vi "输入数据解析.vi"(0 "单个参数补充":dbl, 1 "从板号":dbl=1.0, 2 "主板二维码":string="BNET01", 3 "从板二维码":string="BNET01", 5 "主板引用":refnum<vi>, 7 "从板引用":refnum<vi>, 9 "主板选项":string="三级故障阀值", 11 "枚举":enum16{"主板", "从板"}(ring), 12 "快换":bool caption="快换写入") -> (4 "输出数组":dbl[][](array[numeric]), 6 "数组长度":dbl[](array[numeric]), 8 "循环次数":i32, 10 "命令":u32, 14 "名称":string[](array[string]), 15 "命令序号":u32[](array[numeric]))   [LabVIEW 2013] (continued)
                  disable-tunnel: [w8295 255 ("高字节1")] -> w8291
                  disable-tunnel: w8289 -> [w8293 _]
                  frame Disabled {
                    n3202 = Unbundle By Name(w8293) -> ("单组温度不均衡"=w8292:dbl)
                    n3203 = call "输入分辨率计算-EV05.vi"("1字节?"=TRUE, "数值"=w8292, "偏移量"=0.0, "分辨率"=1.0) -> ("高字节1"=w8295:dbl)  [unwired: 1 in, 6 out]
                  }
                  frame Enabled {
                  }
                }
                n3204 = Build Array(w8291) -> (w8290:i32[])
              }
              frame 12 {
                n3205 = Unbundle By Name(w8303) -> ("SOC过高"=w8302:dbl)
                n3206 = call "输入分辨率计算-EV05.vi"("1字节?"=FALSE, "数值"=w8302, "偏移量"=0.0, "分辨率"=0.1) -> ("低字节"=w8304:dbl, "高字节1"=w8305:dbl)  [unwired: 1 in, 5 out]
                n3207 = call "二进制解析-8.6.vi"("索引"=4, "数值"=w8305) -> ("低位子数组"=w8308:i32[])  [unwired: 3 out]
                n3208 = call "二进制解析-8.6.vi"("索引"=4, "数值"=w8304) -> ("低位子数组"=w8300:i32[], "高位子数组"=w8307:i32[])  [unwired: 2 out]
                n3209 = Insert Into Array(array=w8308, new element=w8307) -> (w8306:i32[])  [unwired: 1 in]
                n3210 = call "数值二进制转十进制-8.6.vi"("子数组"=w8306) -> ("十进制数值"=w8301:i32)  [unwired: 4 out]
                n3211 = disable-structure shown="启用" {
                  disable-tunnel: w8301 -> [w8316 _]
                  disable-tunnel: [w8316 255 ("高字节1")] -> w8299
                  disable-tunnel: [w8315 i32[] [] ("低位子数组 28")] -> _
                  disable-tunnel: w8300 -> [w8315 _]
                  frame Disabled {
                  }
                  frame Enabled {
                  }
                }
                n3212 = Build Array(w8299, w8299) -> (w8312:i32[])
              }
              frame 13 {
                # "SOC过低"
                n3213 = Unbundle By Name(w8324) -> ("SOC过低"=w8323:dbl)
                n3214 = call "输入分辨率计算-EV05.vi"("1字节?"=FALSE, "数值"=w8323, "偏移量"=0.0, "分辨率"=0.1) -> ("低字节"=w8321:dbl, "高字节1"=w8322:dbl)  [unwired: 1 in, 5 out]
                n3215 = call "二进制解析-8.6.vi"("索引"=4, "数值"=w8322) -> ("低位子数组"=w8320:i32[])  [unwired: 3 out]
                n3216 = disable-structure shown="启用" {
                  disable-tunnel: w8321 -> [w8331 _]
                  disable-tunnel: [w8331 255 ("高字节1")] -> w8319
                  disable-tunnel: w8320 -> [w8330 _]
                  disable-tunnel: [w8330 i32[] [] ("低位子数组")] -> _
                  frame Disabled {
                    (unwired) i32[] [] ("低位子数组 4")
                  }
                  frame Enabled {
                  }
                }
                n3217 = Build Array(w8319, w8319) -> (w8327:i32[])
              }
              frame 14 {
                # "内阻过大"
                n3218 = disable-structure shown="启用" {
                  disable-tunnel: w8336 -> [w8341 _]
                  disable-tunnel: [w8337 255 ("高字节1")] -> w8334
                  frame Disabled {
                    n3219 = Unbundle By Name(w8341) -> ("内阻过大"=w8340:dbl)
                    n3220 = call "输入分辨率计算-EV05.vi"("1字节?"=TRUE, "数值"=w8340, "分辨率"=0.1) -> ("高字节1"=w8337:dbl)  [unwired: 2 in, 6 out]
                  }
                  frame Enabled {
                  }
                }
                n3221 = Build Array(w8334) -> (w8335:i32[])
              }
              frame 15 {
                # "极柱温度过高"
                n3222 = disable-structure shown="启用" {
                  disable-tunnel: w8345 -> [w8351 _]
                  disable-tunnel: [w8347 255 ("高字节1")] -> w8343
                  frame Disabled {
                    n3223 = Unbundle By Name(w8351) -> ("极柱温度过高"=w8350:dbl)
                    n3224 = call "输入分辨率计算-EV05.vi"("1字节?"=TRUE, "数值"=w8350, "偏移量"=-40.0, "分辨率"=1.0) -> ("高字节1"=w8347:dbl)  [unwired: 1 in, 6 out]
                  }
                  frame Enabled {
                  }
                }
                n3225 = Build Array(w8343) -> (w8344:i32[])
              }
              frame 16 {
                # "SOH过低"
                n3226 = disable-structure shown="启用" {
                  disable-tunnel: [w8368 w8376] -> w8355
                  disable-tunnel: w8354 -> [w8365 _]
                  disable-tunnel: [w8357 w8376] -> w8353
                  frame Disabled {
                    n3227 = Unbundle By Name(w8365) -> ("SOH过低"=w8364:dbl)
                    n3228 = call "输入分辨率计算-EV05.vi"("1字节?"=FALSE, "数值"=w8364, "偏移量"=0.0, "分辨率"=0.1) -> ("低字节"=w8366:dbl, "高字节1"=w8367:dbl)  [unwired: 1 in, 5 out]
                    n3229 = call "二进制解析-8.6.vi"("索引"=4, "数值"=w8367) -> ("低位子数组"=w8370:i32[])  [unwired: 3 out]
                    n3230 = call "二进制解析-8.6.vi"("索引"=4, "数值"=w8366) -> ("低位子数组"=w8359:i32[], "高位子数组"=w8369:i32[])  [unwired: 2 out]
                    n3231 = call "二进制解析-8.6.vi"("索引"=4, "数值"=0) -> ("低位子数组"=w8360:i32[])  [unwired: 3 out]
                    n3232 = Insert Into Array(array=w8370, new element=w8369) -> (w8363:i32[])  [unwired: 1 in]
                    n3233 = Insert Into Array(array=w8359, new element=w8360) -> (w8358:i32[])  [unwired: 1 in]
                    n3234 = call "数值二进制转十进制-8.6.vi"("子数组"=w8363) -> ("十进制数值"=w8368:i32)  [unwired: 4 out]
                    n3235 = call "数值二进制转十进制-8.6.vi"("子数组"=w8358) -> ("十进制数值"=w8357:i32)  [unwired: 4 out]
                  }
                  frame Enabled {
                    w8376 = 255 ("高字节1")
                  }
                }
                n3236 = Build Array(w8355, w8353) -> (w8356:i32[])
              }
            }
            n3237 = Insert Into Array(array=w8161, new element=w8162) -> (w8160:dbl[])  [unwired: 1 in]
          }
          n3238 = Build Array(w8157) -> (w8156:dbl[][])
          n3239 = Build Array("二级故障阀值") -> (w8147:string[])
        }
        frame "放电电流过高(3)" {
          n3240 = Unbundle By Name(w8382) -> ("一级故障 3"=w8383:refnum<vi>)
          n3241 = property class="Clust (严格)"(reference=w8383) -> ("Value"=w8381:T4)  [unwired: 1 in, 2 out]
          n3242 = for {
            N: 17 -> [_]
            tunnel: w8381 -> [w8393]
            shift-right: [w8390] -> w8387
            shift-left: dbl[] [] -> [w8391]
            i -> [w8394]
            n3243 = case shown="14" w8394 {
              tunnel: w8393 -> [w8395 w8406 w8417 w8427 w8437 w8447 w8459 w8471 w8483 w8495 w8507 w8519 w8533 w8554 w8566 w8575 w8584]
              tunnel: [w8396 w8407 w8418 w8428 w8438 w8449 w8461 w8473 w8485 w8497 w8509 w8520 w8542 w8557 w8565 w8574 w8586] -> w8392
              frame 0, Default {
                # "总电压过高"
                n3244 = disable-structure shown="启用" {
                  disable-tunnel: [w8402 w8405] -> w8398
                  disable-tunnel: [w8401 w8405] -> w8397
                  disable-tunnel: w8395 -> [w8400 _]
                  frame Disabled {
                    n3245 = Unbundle By Name(w8400) -> ("总电压过高"=w8399:dbl)
                    n3246 = call "输入分辨率计算-EV05.vi"("1字节?"=FALSE, "数值"=w8399, "分辨率"=0.1) -> ("低字节"=w8402:dbl, "高字节1"=w8401:dbl)  [unwired: 2 in, 5 out]
                  }
                  frame Enabled {
                    w8405 = 255 ("高字节1")
                  }
                }
                n3247 = Build Array(w8397, w8398) -> (w8396:i32[])
              }
              frame 1 {
                # "总电压过低"
                n3248 = disable-structure shown="启用" {
                  disable-tunnel: [w8413 w8416] -> w8409
                  disable-tunnel: [w8412 w8416] -> w8408
                  disable-tunnel: w8406 -> [w8411 _]
                  frame Disabled {
                    n3249 = Unbundle By Name(w8411) -> ("总电压过低"=w8410:dbl)
                    n3250 = call "输入分辨率计算-EV05.vi"("1字节?"=FALSE, "数值"=w8410, "分辨率"=0.1) -> ("低字节"=w8413:dbl, "高字节1"=w8412:dbl)  [unwired: 2 in, 5 out]
                  }
                  frame Enabled {
                    w8416 = 255 ("高字节1")
                  }
                }
                n3251 = Build Array(w8408, w8409) -> (w8407:i32[])
              }
              frame 2 {
                # "温度过高"
                n3252 = disable-structure shown="启用" {
                  disable-tunnel: [w8423 255 ("高字节1")] -> w8419
                  disable-tunnel: w8417 -> [w8421 _]
                  frame Disabled {
                    n3253 = Unbundle By Name(w8421) -> ("温度过高"=w8420:dbl)
                    n3254 = call "输入分辨率计算-EV05.vi"("1字节?"=TRUE, "数值"=w8420, "偏移量"=-40.0, "分辨率"=1.0) -> ("高字节1"=w8423:dbl)  [unwired: 1 in, 6 out]
                  }
                  frame Enabled {
                  }
                }
                n3255 = Build Array(w8419) -> (w8418:i32[])
              }
              frame 3 {
                # "温度过低"
                n3256 = disable-structure shown="启用" {
                  disable-tunnel: [w8433 255 ("高字节1")] -> w8429
                  disable-tunnel: w8427 -> [w8431 _]
                  frame Disabled {
                    n3257 = Unbundle By Name(w8431) -> ("温度过低"=w8430:dbl)
                    n3258 = call "输入分辨率计算-EV05.vi"("1字节?"=TRUE, "数值"=w8430, "偏移量"=-40.0, "分辨率"=1.0) -> ("高字节1"=w8433:dbl)  [unwired: 1 in, 6 out]
                  }
                  frame Enabled {
                  }
                }
                n3259 = Build Array(w8429) -> (w8428:i32[])
              }
              frame 4 {
                # "整组温度不均衡"
                n3260 = disable-structure shown="启用" {
                  disable-tunnel: [w8443 255 ("高字节1")] -> w8439
                  disable-tunnel: w8437 -> [w8441 _]
                  frame Disabled {
                    n3261 = Unbundle By Name(w8441) -> ("整组温度不均衡"=w8440:dbl)
                    n3262 = call "输入分辨率计算-EV05.vi"("1字节?"=TRUE, "数值"=w8440, "偏移量"=0.0, "分辨率"=1.0) -> ("高字节1"=w8443:dbl)  [unwired: 1 in, 6 out]
                  }
                  frame Enabled {
                  }
                }
                n3263 = Build Array(w8439) -> (w8438:i32[])
              }
              frame 5 {
                # "单组电压不均衡"
                n3264 = disable-structure shown="启用" {
                  disable-tunnel: [w8455 w8458] -> w8450
                  disable-tunnel: [w8453 w8458] -> w8448
                  disable-tunnel: w8447 -> [w8452 _]
                  frame Disabled {
                    n3265 = Unbundle By Name(w8452) -> ("单组电压不均衡"=w8451:dbl)
                    n3266 = call "输入分辨率计算-EV05.vi"("1字节?"=FALSE, "数值"=w8451, "偏移量"=0.0, "分辨率"=0.001) -> ("低字节"=w8453:dbl, "高字节1"=w8455:dbl)  [unwired: 1 in, 5 out]
                  }
                  frame Enabled {
                    w8458 = 255 ("高字节1")
                  }
                }
                n3267 = Build Array(w8450, w8448) -> (w8449:i32[])
              }
              frame 6 {
                # "整组电压不均衡"
                n3268 = disable-structure shown="启用" {
                  disable-tunnel: [w8467 w8470] -> w8462
                  disable-tunnel: [w8465 w8470] -> w8460
                  disable-tunnel: w8459 -> [w8464 _]
                  frame Disabled {
                    n3269 = Unbundle By Name(w8464) -> ("整组电压不均衡"=w8463:dbl)
                    n3270 = call "输入分辨率计算-EV05.vi"("1字节?"=FALSE, "数值"=w8463, "偏移量"=0.0, "分辨率"=0.001) -> ("低字节"=w8465:dbl, "高字节1"=w8467:dbl)  [unwired: 1 in, 5 out]
                  }
                  frame Enabled {
                    w8470 = 255 ("高字节1")
                  }
                }
                n3271 = Build Array(w8462, w8460) -> (w8461:i32[])
              }
              frame 7 {
                # "单体电压过高"
                n3272 = disable-structure shown="启用" {
                  disable-tunnel: [w8479 w8482] -> w8474
                  disable-tunnel: [w8477 w8482] -> w8472
                  disable-tunnel: w8471 -> [w8476 _]
                  frame Disabled {
                    n3273 = Unbundle By Name(w8476) -> ("单体电压过高"=w8475:dbl)
                    n3274 = call "输入分辨率计算-EV05.vi"("1字节?"=FALSE, "数值"=w8475, "偏移量"=0.0, "分辨率"=0.001) -> ("低字节"=w8477:dbl, "高字节1"=w8479:dbl)  [unwired: 1 in, 5 out]
                  }
                  frame Enabled {
                    w8482 = 255 ("高字节1")
                  }
                }
                n3275 = Build Array(w8474, w8472) -> (w8473:i32[])
              }
              frame 8 {
                # "单体电压过低"
                n3276 = disable-structure shown="启用" {
                  disable-tunnel: [w8491 w8494] -> w8486
                  disable-tunnel: [w8489 w8494] -> w8484
                  disable-tunnel: w8483 -> [w8488 _]
                  frame Disabled {
                    n3277 = Unbundle By Name(w8488) -> ("单体电压过低"=w8487:dbl)
                    n3278 = call "输入分辨率计算-EV05.vi"("1字节?"=FALSE, "数值"=w8487, "偏移量"=0.0, "分辨率"=0.001) -> ("低字节"=w8489:dbl, "高字节1"=w8491:dbl)  [unwired: 1 in, 5 out]
                  }
                  frame Enabled {
                    w8494 = 255 ("高字节1")
                  }
                }
                n3279 = Build Array(w8486, w8484) -> (w8485:i32[])
              }
              frame 9 {
                # "充电电流过高"
                n3280 = disable-structure shown="启用" {
                  disable-tunnel: [w8503 w8506] -> w8498
                  disable-tunnel: [w8501 w8506] -> w8496
                  disable-tunnel: w8495 -> [w8500 _]
                  frame Disabled {
                    n3281 = Unbundle By Name(w8500) -> ("充电电流过高"=w8499:dbl)
                    n3282 = call "输入分辨率计算-EV05.vi"("1字节?"=FALSE, "数值"=w8499, "偏移量"=-3000.0, "分辨率"=0.1) -> ("低字节"=w8501:dbl, "高字节1"=w8503:dbl)  [unwired: 1 in, 5 out]
                  }
                  frame Enabled {
                    w8506 = 255 ("高字节1")
                  }
                }
                n3283 = Build Array(w8498, w8496) -> (w8497:i32[])
              }
              frame 10 {
                # "放电电流过高"
                n3284 = disable-structure shown="启用" {
                  disable-tunnel: [w8515 w8518] -> w8510
                  disable-tunnel: [w8513 w8518] -> w8508
                  disable-tunnel: w8507 -> [w8512 _]
                  frame Enabled {
                    n3285 = Unbundle By Name(w8512) -> ("放电电流过高"=w8511:dbl)
                    n3286 = call "输入分辨率计算-EV05.vi"("1字节?"=FALSE, "数值"=w8511, "偏移量"=0.0, "分辨率"=0.1) -> ("低字节"=w8513:dbl, "高字节1"=w8515:dbl)  [unwired: 1 in, 5 out]
                  }
                  frame Disabled {
                    w8518 = 255 ("高字节1")
                  }
                }
                n3287 = Build Array(w8510, w8508) -> (w8509:dbl[])
              }
              frame 11 {
                # "单组温度不均衡"
                n3288 = disable-structure shown="启用" {
                  disable-tunnel: [w8525 255 ("高字节1")] -> w8521
                  disable-tunnel: w8519 -> [w8523 _]
                  frame Disabled {
                    n3289 = Unbundle By Name(w8523) -> ("单组温度不均衡"=w8522:dbl)
                    n3290 = call "输入分辨率计算-EV05.vi"("1字节?"=TRUE, "数值"=w8522, "偏移量"=0.0, "分辨率"=1.0) -> ("高字节1"=w8525:dbl)  [unwired: 1 in, 6 out]
                  }
                  frame Enabled {
                  }
                }
                n3291 = Build Array(w8521) -> (w8520:i32[])
              }
              frame 12 {
                # "SOC过高"
                n3292 = Unbundle By Name(w8533) -> ("SOC过高"=w8532:dbl)
                n3293 = call "输入分辨率计算-EV05.vi"("1字节?"=FALSE, "数值"=w8532, "偏移量"=0.0, "分辨率"=0.1) -> ("低字节"=w8534:dbl, "高字节1"=w8535:dbl)  [unwired: 1 in, 5 out]
                n3294 = call "二进制解析-8.6.vi"("索引"=4, "数值"=w8535) -> ("低位子数组"=w8538:i32[])  [unwired: 3 out]
                n3295 = call "二进制解析-8.6.vi"("索引"=4, "数值"=w8534) -> ("低位子数组"=w8530:i32[], "高位子数组"=w8537:i32[])  [unwired: 2 out]
                n3296 = Insert Into Array(array=w8538, new element=w8537) -> (w8536:i32[])  [unwired: 1 in]
                n3297 = call "数值二进制转十进制-8.6.vi"("子数组"=w8536) -> ("十进制数值"=w8531:i32)  [unwired: 4 out]
                n3298 = disable-structure shown="启用" {
                  disable-tunnel: w8531 -> [w8546 _]
                  disable-tunnel: [w8546 255 ("高字节1")] -> w8529
                  disable-tunnel: [w8545 i32[] [] ("低位子数组 28")] -> _
                  disable-tunnel: w8530 -> [w8545 _]
                  frame Disabled {
                  }
                  frame Enabled {
                  }
                }
                n3299 = Build Array(w8529, w8529) -> (w8542:i32[])
              }
              frame 13 {
                # "SOC过低"
                n3300 = Unbundle By Name(w8554) -> ("SOC过低"=w8553:dbl)
                n3301 = call "输入分辨率计算-EV05.vi"("1字节?"=FALSE, "数值"=w8553, "偏移量"=0.0, "分辨率"=0.1) -> ("低字节"=w8551:dbl, "高字节1"=w8552:dbl)  [unwired: 1 in, 5 out]
                n3302 = call "二进制解析-8.6.vi"("索引"=4, "数值"=w8552) -> ("低位子数组"=w8550:i32[])  [unwired: 3 out]
                n3303 = disable-structure shown="启用" {
                  disable-tunnel: w8551 -> [w8561 _]
                  disable-tunnel: [w8561 255 ("高字节1")] -> w8549
                  disable-tunnel: w8550 -> [w8560 _]
                  disable-tunnel: [w8560 i32[] [] ("低位子数组")] -> _
                  frame Disabled {
                    (unwired) i32[] [] ("低位子数组 4")
                  }
                  frame Enabled {
                  }
                }
                n3304 = Build Array(w8549, w8549) -> (w8557:i32[])
              }
              frame 14 {
                # "内阻过大"
                n3305 = disable-structure shown="启用" {
                  disable-tunnel: w8566 -> [w8571 _]
                  disable-tunnel: [w8567 255 ("高字节1")] -> w8564
                  frame Disabled {
                    n3306 = Unbundle By Name(w8571) -> ("内阻过大"=w8570:dbl)
                    n3307 = call "输入分辨率计算-EV05.vi"("1字节?"=TRUE, "数值"=w8570, "分辨率"=0.1) -> ("高字节1"=w8567:dbl)  [unwired: 2 in, 6 out]
                  }
                  frame Enabled {
                  }
                }
                n3308 = Build Array(w8564) -> (w8565:i32[])
              }
              frame 15 {
                # "极柱温度过高"
                n3309 = disable-structure shown="启用" {
                  disable-tunnel: w8575 -> [w8581 _]
                  disable-tunnel: [w8577 255 ("高字节1")] -> w8573
                  frame Disabled {
                    n3310 = Unbundle By Name(w8581) -> ("极柱温度过高"=w8580:dbl)
                    n3311 = call "输入分辨率计算-EV05.vi"("1字节?"=TRUE, "数值"=w8580, "偏移量"=-40.0, "分辨率"=1.0) -> ("高字节1"=w8577:dbl)  [unwired: 1 in, 6 out]
                  }
                  frame Enabled {
                  }
                }
                n3312 = Build Array(w8573) -> (w8574:i32[])
              }
              frame 16 {
                # "SOH过低"
                n3313 = disable-structure shown="启用" {
                  disable-tunnel: [w8598 w8606] -> w8585
                  disable-tunnel: w8584 -> [w8595 _]
                  disable-tunnel: [w8587 w8606] -> w8583
                  frame Disabled {
                    n3314 = Unbundle By Name(w8595) -> ("SOH过低"=w8594:dbl)
                    n3315 = call "输入分辨率计算-EV05.vi"("1字节?"=FALSE, "数值"=w8594, "偏移量"=0.0, "分辨率"=0.1) -> ("低字节"=w8596:dbl, "高字节1"=w8597:dbl)  [unwired: 1 in, 5 out]
                    n3316 = call "二进制解析-8.6.vi"("索引"=4, "数值"=w8597) -> ("低位子数组"=w8600:i32[])  [unwired: 3 out]
                    n3317 = call "二进制解析-8.6.vi"("索引"=4, "数值"=w8596) -> ("低位子数组"=w8589:i32[], "高位子数组"=w8599:i32[])  [unwired: 2 out]
                    n3318 = call "二进制解析-8.6.vi"("索引"=4, "数值"=0) -> ("低位子数组"=w8590:i32[])  [unwired: 3 out]
                    n3319 = Insert Into Array(array=w8600, new element=w8599) -> (w8593:i32[])  [unwired: 1 in]
                    n3320 = Insert Into Array(array=w8589, new element=w8590) -> (w8588:i32[])  [unwired: 1 in]
                    n3321 = call "数值二进制转十进制-8.6.vi"("子数组"=w8593) -> ("十进制数值"=w8598:i32)  [unwired: 4 out]
                    n3322 = call "数值二进制转十进制-8.6.vi"("子数组"=w8588) -> ("十进制数值"=w8587:i32)  [unwired: 4 out]
                  }
                  frame Enabled {
                    w8606 = 255 ("高字节1")
                  }
                }
                n3323 = Build Array(w8585, w8583) -> (w8586:i32[])
              }
            }
            n3324 = Insert Into Array(array=w8391, new element=w8392) -> (w8390:dbl[])  [unwired: 1 in]
          }
          n3325 = Build Array(w8387) -> (w8386:dbl[][])
          n3326 = Build Array("三级故障阀值") -> (w8377:string[])
        }
        frame "单组温度不均衡" {
          n3327 = Unbundle By Name(w8612) -> ("一级故障"=w8613:refnum<vi>)
          n3328 = property class="Clust (严格)"(reference=w8613) -> ("Value"=w8611:T4)  [unwired: 1 in, 2 out]
          n3329 = for {
            N: 17 -> [_]
            tunnel: w8611 -> [w8623]
            shift-right: [w8620] -> w8617
            shift-left: dbl[] [] -> [w8621]
            i -> [w8624]
            n3330 = case shown="11" w8624 {
              tunnel: w8623 -> [w8625 w8636 w8647 w8657 w8667 w8677 w8689 w8701 w8713 w8725 w8737 w8749 w8762 w8783 w8795 w8804 w8813]
              tunnel: [w8626 w8637 w8648 w8658 w8668 w8679 w8691 w8703 w8715 w8727 w8739 w8750 w8771 w8786 w8794 w8803 w8815] -> w8622
              frame 0, Default {
                # "总电压过高"
                n3331 = disable-structure shown="启用" {
                  disable-tunnel: [w8632 w8635] -> w8628
                  disable-tunnel: [w8631 w8635] -> w8627
                  disable-tunnel: w8625 -> [w8630 _]
                  frame Disabled {
                    n3332 = Unbundle By Name(w8630) -> ("总电压过高"=w8629:dbl)
                    n3333 = call "输入分辨率计算-EV05.vi"("1字节?"=FALSE, "数值"=w8629, "分辨率"=0.1) -> ("低字节"=w8632:dbl, "高字节1"=w8631:dbl)  [unwired: 2 in, 5 out]
                  }
                  frame Enabled {
                    w8635 = 255 ("高字节1")
                  }
                }
                n3334 = Build Array(w8627, w8628) -> (w8626:i32[])
              }
              frame 1 {
                # "总电压过低"
                n3335 = disable-structure shown="启用" {
                  disable-tunnel: [w8643 w8646] -> w8639
                  disable-tunnel: [w8642 w8646] -> w8638
                  disable-tunnel: w8636 -> [w8641 _]
                  frame Disabled {
                    n3336 = Unbundle By Name(w8641) -> ("总电压过低"=w8640:dbl)
                    n3337 = call "输入分辨率计算-EV05.vi"("1字节?"=FALSE, "数值"=w8640, "分辨率"=0.1) -> ("低字节"=w8643:dbl, "高字节1"=w8642:dbl)  [unwired: 2 in, 5 out]
                  }
                  frame Enabled {
                    w8646 = 255 ("高字节1")
                  }
                }
                n3338 = Build Array(w8638, w8639) -> (w8637:i32[])
              }
              frame 2 {
                # "温度过高"
                n3339 = disable-structure shown="启用" {
                  disable-tunnel: [w8653 255 ("高字节1")] -> w8649
                  disable-tunnel: w8647 -> [w8651 _]
                  frame Disabled {
                    n3340 = Unbundle By Name(w8651) -> ("温度过高"=w8650:dbl)
                    n3341 = call "输入分辨率计算-EV05.vi"("1字节?"=TRUE, "数值"=w8650, "偏移量"=-40.0, "分辨率"=1.0) -> ("高字节1"=w8653:dbl)  [unwired: 1 in, 6 out]
                  }
                  frame Enabled {
                  }
                }
                n3342 = Build Array(w8649) -> (w8648:i32[])
              }
              frame 3 {
                # "温度过低"
                n3343 = disable-structure shown="启用" {
                  disable-tunnel: [w8663 255 ("高字节1")] -> w8659
                  disable-tunnel: w8657 -> [w8661 _]
                  frame Disabled {
                    n3344 = Unbundle By Name(w8661) -> ("温度过低"=w8660:dbl)
                    n3345 = call "输入分辨率计算-EV05.vi"("1字节?"=TRUE, "数值"=w8660, "偏移量"=-40.0, "分辨率"=1.0) -> ("高字节1"=w8663:dbl)  [unwired: 1 in, 6 out]
                  }
                  frame Enabled {
                  }
                }
                n3346 = Build Array(w8659) -> (w8658:i32[])
              }
              frame 4 {
                # "整组温度不均衡"
                n3347 = disable-structure shown="启用" {
                  disable-tunnel: [w8673 255 ("高字节1")] -> w8669
                  disable-tunnel: w8667 -> [w8671 _]
                  frame Disabled {
                    n3348 = Unbundle By Name(w8671) -> ("整组温度不均衡"=w8670:dbl)
                    n3349 = call "输入分辨率计算-EV05.vi"("1字节?"=TRUE, "数值"=w8670, "偏移量"=0.0, "分辨率"=1.0) -> ("高字节1"=w8673:dbl)  [unwired: 1 in, 6 out]
                  }
                  frame Enabled {
                  }
                }
                n3350 = Build Array(w8669) -> (w8668:i32[])
              }
              frame 5 {
                # "单组电压不均衡"
                n3351 = disable-structure shown="启用" {
                  disable-tunnel: [w8685 w8688] -> w8680
                  disable-tunnel: [w8683 w8688] -> w8678
                  disable-tunnel: w8677 -> [w8682 _]
                  frame Disabled {
                    n3352 = Unbundle By Name(w8682) -> ("单组电压不均衡"=w8681:dbl)
                    n3353 = call "输入分辨率计算-EV05.vi"("1字节?"=FALSE, "数值"=w8681, "偏移量"=0.0, "分辨率"=0.001) -> ("低字节"=w8683:dbl, "高字节1"=w8685:dbl)  [unwired: 1 in, 5 out]
                  }
                  frame Enabled {
                    w8688 = 255 ("高字节1")
                  }
                }
                n3354 = Build Array(w8680, w8678) -> (w8679:i32[])
              }
              frame 6 {
                # "整组电压不均衡"
                n3355 = disable-structure shown="启用" {
                  disable-tunnel: [w8697 w8700] -> w8692
                  disable-tunnel: [w8695 w8700] -> w8690
                  disable-tunnel: w8689 -> [w8694 _]
                  frame Disabled {
                    n3356 = Unbundle By Name(w8694) -> ("整组电压不均衡"=w8693:dbl)
                    n3357 = call "输入分辨率计算-EV05.vi"("1字节?"=FALSE, "数值"=w8693, "偏移量"=0.0, "分辨率"=0.001) -> ("低字节"=w8695:dbl, "高字节1"=w8697:dbl)  [unwired: 1 in, 5 out]
                  }
                  frame Enabled {
                    w8700 = 255 ("高字节1")
                  }
                }
                n3358 = Build Array(w8692, w8690) -> (w8691:i32[])
              }
              frame 7 {
                # "单体电压过高"
                n3359 = disable-structure shown="启用" {
                  disable-tunnel: [w8709 w8712] -> w8704
                  disable-tunnel: [w8707 w8712] -> w8702
                  disable-tunnel: w8701 -> [w8706 _]
                  frame Disabled {
                    n3360 = Unbundle By Name(w8706) -> ("单体电压过高"=w8705:dbl)
                    n3361 = call "输入分辨率计算-EV05.vi"("1字节?"=FALSE, "数值"=w8705, "偏移量"=0.0, "分辨率"=0.001) -> ("低字节"=w8707:dbl, "高字节1"=w8709:dbl)  [unwired: 1 in, 5 out]
                  }
                  frame Enabled {
                    w8712 = 255 ("高字节1")
                  }
                }
                n3362 = Build Array(w8704, w8702) -> (w8703:i32[])
              }
              frame 8 {
                # "单体电压过低"
                n3363 = disable-structure shown="启用" {
                  disable-tunnel: [w8721 w8724] -> w8716
                  disable-tunnel: [w8719 w8724] -> w8714
                  disable-tunnel: w8713 -> [w8718 _]
                  frame Disabled {
                    n3364 = Unbundle By Name(w8718) -> ("单体电压过低"=w8717:dbl)
                    n3365 = call "输入分辨率计算-EV05.vi"("1字节?"=FALSE, "数值"=w8717, "偏移量"=0.0, "分辨率"=0.001) -> ("低字节"=w8719:dbl, "高字节1"=w8721:dbl)  [unwired: 1 in, 5 out]
                  }
                  frame Enabled {
                    w8724 = 255 ("高字节1")
                  }
                }
                n3366 = Build Array(w8716, w8714) -> (w8715:i32[])
              }
              frame 9 {
                # "充电电流过高"
                n3367 = disable-structure shown="启用" {
                  disable-tunnel: [w8733 w8736] -> w8728
                  disable-tunnel: [w8731 w8736] -> w8726
                  disable-tunnel: w8725 -> [w8730 _]
                  frame Disabled {
                    n3368 = Unbundle By Name(w8730) -> ("充电电流过高"=w8729:dbl)
                    n3369 = call "输入分辨率计算-EV05.vi"("1字节?"=FALSE, "数值"=w8729, "偏移量"=-3000.0, "分辨率"=0.1) -> ("低字节"=w8731:dbl, "高字节1"=w8733:dbl)  [unwired: 1 in, 5 out]
                  }
                  frame Enabled {
                    w8736 = 255 ("高字节1")
                  }
                }
                n3370 = Build Array(w8728, w8726) -> (w8727:i32[])
              }
              frame 10 {
                # "放电电流过高"
                n3371 = disable-structure shown="启用" {
                  disable-tunnel: [w8745 w8748] -> w8740
                  disable-tunnel: [w8743 w8748] -> w8738
                  disable-tunnel: w8737 -> [w8742 _]
                  frame Disabled {
                    n3372 = Unbundle By Name(w8742) -> ("放电电流过高"=w8741:dbl)
                    n3373 = call "输入分辨率计算-EV05.vi"("1字节?"=FALSE, "数值"=w8741, "偏移量"=-3000.0, "分辨率"=0.1) -> ("低字节"=w8743:dbl, "高字节1"=w8745:dbl)  [unwired: 1 in, 5 out]
                  }
                  frame Enabled {
                    w8748 = 255 ("高字节1")
                  }
                }
                n3374 = Build Array(w8740, w8738) -> (w8739:i32[])
              }
              frame 11 {
                # "单组温度不均衡"
                n3375 = disable-structure shown="启用" {
                  disable-tunnel: [w8754 255 ("高字节1")] -> w8751
                  disable-tunnel: w8749 -> [w8753 _]
                  frame Enabled {
                    n3376 = Unbundle By Name(w8753) -> ("单组温度不均衡"=w8752:dbl)
                    n3377 = call "输入分辨率计算-EV05.vi"("1字节?"=TRUE, "数值"=w8752, "分辨率"=1.0) -> ("高字节1"=w8754:dbl)  [unwired: 2 in, 6 out]
                  }
                  frame Disabled {
                  }
                }
                n3378 = Build Array(w8751) -> (w8750:dbl[])
              }
              frame 12 {
                # "SOC过高"
                n3379 = Unbundle By Name(w8762) -> ("SOC过高"=w8761:dbl)
                n3380 = call "输入分辨率计算-EV05.vi"("1字节?"=FALSE, "数值"=w8761, "偏移量"=0.0, "分辨率"=0.1) -> ("低字节"=w8763:dbl, "高字节1"=w8764:dbl)  [unwired: 1 in, 5 out]
                n3381 = call "二进制解析-8.6.vi"("索引"=4, "数值"=w8764) -> ("低位子数组"=w8767:i32[])  [unwired: 3 out]
                n3382 = call "二进制解析-8.6.vi"("索引"=4, "数值"=w8763) -> ("低位子数组"=w8759:i32[], "高位子数组"=w8766:i32[])  [unwired: 2 out]
                n3383 = Insert Into Array(array=w8767, new element=w8766) -> (w8765:i32[])  [unwired: 1 in]
                n3384 = call "数值二进制转十进制-8.6.vi"("子数组"=w8765) -> ("十进制数值"=w8760:i32)  [unwired: 4 out]
                n3385 = disable-structure shown="启用" {
                  disable-tunnel: w8760 -> [w8775 _]
                  disable-tunnel: [w8775 255 ("高字节1")] -> w8758
                  disable-tunnel: w8759 -> [w8774 _]
                  disable-tunnel: [w8774 i32[] [] ("低位子数组 29")] -> _
                  frame Disabled {
                  }
                  frame Enabled {
                  }
                }
                n3386 = Build Array(w8758, w8758) -> (w8771:i32[])
              }
              frame 13 {
                # "SOC过低"
                n3387 = Unbundle By Name(w8783) -> ("SOC过低"=w8782:dbl)
                n3388 = call "输入分辨率计算-EV05.vi"("1字节?"=FALSE, "数值"=w8782, "偏移量"=0.0, "分辨率"=0.1) -> ("低字节"=w8780:dbl, "高字节1"=w8781:dbl)  [unwired: 1 in, 5 out]
                n3389 = call "二进制解析-8.6.vi"("索引"=4, "数值"=w8781) -> ("低位子数组"=w8779:i32[])  [unwired: 3 out]
                n3390 = disable-structure shown="启用" {
                  disable-tunnel: w8780 -> [w8790 _]
                  disable-tunnel: [w8790 255 ("高字节1")] -> w8778
                  disable-tunnel: w8779 -> [w8789 _]
                  disable-tunnel: [w8789 i32[] [] ("低位子数组")] -> _
                  frame Disabled {
                    (unwired) i32[] [] ("低位子数组 4")
                  }
                  frame Enabled {
                  }
                }
                n3391 = Build Array(w8778, w8778) -> (w8786:i32[])
              }
              frame 14 {
                # "内阻过大"
                n3392 = disable-structure shown="启用" {
                  disable-tunnel: w8795 -> [w8800 _]
                  disable-tunnel: [w8796 255 ("高字节1")] -> w8793
                  frame Disabled {
                    n3393 = Unbundle By Name(w8800) -> ("内阻过大"=w8799:dbl)
                    n3394 = call "输入分辨率计算-EV05.vi"("1字节?"=TRUE, "数值"=w8799, "分辨率"=0.1) -> ("高字节1"=w8796:dbl)  [unwired: 2 in, 6 out]
                  }
                  frame Enabled {
                  }
                }
                n3395 = Build Array(w8793) -> (w8794:i32[])
              }
              frame 15 {
                # "极柱温度过高"
                n3396 = disable-structure shown="启用" {
                  disable-tunnel: w8804 -> [w8810 _]
                  disable-tunnel: [w8806 255 ("高字节1")] -> w8802
                  frame Disabled {
                    n3397 = Unbundle By Name(w8810) -> ("极柱温度过高"=w8809:dbl)
                    n3398 = call "输入分辨率计算-EV05.vi"("1字节?"=TRUE, "数值"=w8809, "偏移量"=-40.0, "分辨率"=1.0) -> ("高字节1"=w8806:dbl)  [unwired: 1 in, 6 out]
                  }
                  frame Enabled {
                  }
                }
                n3399 = Build Array(w8802) -> (w8803:i32[])
              }
              frame 16 {
                # "SOH过低"
                n3400 = disable-structure shown="启用" {
                  disable-tunnel: [w8827 w8835] -> w8814
                  disable-tunnel: w8813 -> [w8824 _]
                  disable-tunnel: [w8816 w8835] -> w8812
                  frame Disabled {
                    n3401 = Unbundle By Name(w8824) -> ("SOH过低"=w8823:dbl)
                    n3402 = call "输入分辨率计算-EV05.vi"("1字节?"=FALSE, "数值"=w8823, "偏移量"=0.0, "分辨率"=0.1) -> ("低字节"=w8825:dbl, "高字节1"=w8826:dbl)  [unwired: 1 in, 5 out]
                    n3403 = call "二进制解析-8.6.vi"("索引"=4, "数值"=w8826) -> ("低位子数组"=w8829:i32[])  [unwired: 3 out]
                    n3404 = call "二进制解析-8.6.vi"("索引"=4, "数值"=w8825) -> ("低位子数组"=w8818:i32[], "高位子数组"=w8828:i32[])  [unwired: 2 out]
                    n3405 = call "二进制解析-8.6.vi"("索引"=4, "数值"=0) -> ("低位子数组"=w8819:i32[])  [unwired: 3 out]
                    n3406 = Insert Into Array(array=w8829, new element=w8828) -> (w8822:i32[])  [unwired: 1 in]
                    n3407 = Insert Into Array(array=w8818, new element=w8819) -> (w8817:i32[])  [unwired: 1 in]
                    n3408 = call "数值二进制转十进制-8.6.vi"("子数组"=w8822) -> ("十进制数值"=w8827:i32)  [unwired: 4 out]
                    n3409 = call "数值二进制转十进制-8.6.vi"("子数组"=w8817) -> ("十进制数值"=w8816:i32)  [unwired: 4 out]
                  }
                  frame Enabled {
                    w8835 = 255 ("高字节1")
                  }
                }
                n3410 = Build Array(w8814, w8812) -> (w8815:i32[])
              }
            }
            n3411 = Insert Into Array(array=w8621, new element=w8622) -> (w8620:dbl[])  [unwired: 1 in]
          }
          n3412 = Build Array(w8617) -> (w8616:dbl[][])
          n3413 = Build Array("一级故障阀值") -> (w8607:string[])
        }
        frame "单组温度不均衡(2)" {
          n3414 = Unbundle By Name(w8841) -> ("一级故障 2"=w8842:refnum<vi>)
          n3415 = property class="Clust (严格)"(reference=w8842) -> ("Value"=w8840:T4)  [unwired: 1 in, 2 out]
          n3416 = for {
            N: 17 -> [_]
            tunnel: w8840 -> [w8852]
            shift-right: [w8849] -> w8846
            shift-left: dbl[] [] -> [w8850]
            i -> [w8853]
            n3417 = case shown="11" w8853 {
              tunnel: w8852 -> [w8854 w8865 w8876 w8886 w8896 w8906 w8918 w8930 w8942 w8954 w8966 w8978 w8991 w9012 w9024 w9033 w9042]
              tunnel: [w8855 w8866 w8877 w8887 w8897 w8908 w8920 w8932 w8944 w8956 w8968 w8979 w9000 w9015 w9023 w9032 w9044] -> w8851
              frame 0, Default {
                # "总电压过高"
                n3418 = disable-structure shown="启用" {
                  disable-tunnel: [w8861 w8864] -> w8857
                  disable-tunnel: [w8860 w8864] -> w8856
                  disable-tunnel: w8854 -> [w8859 _]
                  frame Disabled {
                    n3419 = Unbundle By Name(w8859) -> ("总电压过高"=w8858:dbl)
                    n3420 = call "输入分辨率计算-EV05.vi"("1字节?"=FALSE, "数值"=w8858, "分辨率"=0.1) -> ("低字节"=w8861:dbl, "高字节1"=w8860:dbl)  [unwired: 2 in, 5 out]
                  }
                  frame Enabled {
                    w8864 = 255 ("高字节1")
                  }
                }
                n3421 = Build Array(w8856, w8857) -> (w8855:i32[])
              }
              frame 1 {
                # "总电压过低"
                n3422 = disable-structure shown="启用" {
                  disable-tunnel: [w8872 w8875] -> w8868
                  disable-tunnel: [w8871 w8875] -> w8867
                  disable-tunnel: w8865 -> [w8870 _]
                  frame Disabled {
                    n3423 = Unbundle By Name(w8870) -> ("总电压过低"=w8869:dbl)
                    n3424 = call "输入分辨率计算-EV05.vi"("1字节?"=FALSE, "数值"=w8869, "分辨率"=0.1) -> ("低字节"=w8872:dbl, "高字节1"=w8871:dbl)  [unwired: 2 in, 5 out]
                  }
                  frame Enabled {
                    w8875 = 255 ("高字节1")
                  }
                }
                n3425 = Build Array(w8867, w8868) -> (w8866:i32[])
              }
              frame 2 {
                # "温度过高"
                n3426 = disable-structure shown="启用" {
                  disable-tunnel: [w8882 255 ("高字节1")] -> w8878
                  disable-tunnel: w8876 -> [w8880 _]
                  frame Disabled {
                    n3427 = Unbundle By Name(w8880) -> ("温度过高"=w8879:dbl)
                    n3428 = call "输入分辨率计算-EV05.vi"("1字节?"=TRUE, "数值"=w8879, "偏移量"=-40.0, "分辨率"=1.0) -> ("高字节1"=w8882:dbl)  [unwired: 1 in, 6 out]
                  }
                  frame Enabled {
                  }
                }
                n3429 = Build Array(w8878) -> (w8877:i32[])
              }
              frame 3 {
                # "温度过低"
                n3430 = disable-structure shown="启用" {
                  disable-tunnel: [w8892 255 ("高字节1")] -> w8888
                  disable-tunnel: w8886 -> [w8890 _]
                  frame Disabled {
                    n3431 = Unbundle By Name(w8890) -> ("温度过低"=w8889:dbl)
                    n3432 = call "输入分辨率计算-EV05.vi"("1字节?"=TRUE, "数值"=w8889, "偏移量"=-40.0, "分辨率"=1.0) -> ("高字节1"=w8892:dbl)  [unwired: 1 in, 6 out]
                  }
                  frame Enabled {
                  }
                }
                n3433 = Build Array(w8888) -> (w8887:i32[])
              }
              frame 4 {
                # "整组温度不均衡"
                n3434 = disable-structure shown="启用" {
                  disable-tunnel: [w8902 255 ("高字节1")] -> w8898
                  disable-tunnel: w8896 -> [w8900 _]
                  frame Disabled {
                    n3435 = Unbundle By Name(w8900) -> ("整组温度不均衡"=w8899:dbl)
                    n3436 = call "输入分辨率计算-EV05.vi"("1字节?"=TRUE, "数值"=w8899, "偏移量"=0.0, "分辨率"=1.0) -> ("高字节1"=w8902:dbl)  [unwired: 1 in, 6 out]
                  }
                  frame Enabled {
                  }
                }
                n3437 = Build Array(w8898) -> (w8897:i32[])
              }
              frame 5 {
                # "单组电压不均衡"
                n3438 = disable-structure shown="启用" {
                  disable-tunnel: [w8914 w8917] -> w8909
                  disable-tunnel: [w8912 w8917] -> w8907
                  disable-tunnel: w8906 -> [w8911 _]
                  frame Disabled {
                    n3439 = Unbundle By Name(w8911) -> ("单组电压不均衡"=w8910:dbl)
                    n3440 = call "输入分辨率计算-EV05.vi"("1字节?"=FALSE, "数值"=w8910, "偏移量"=0.0, "分辨率"=0.001) -> ("低字节"=w8912:dbl, "高字节1"=w8914:dbl)  [unwired: 1 in, 5 out]
                  }
                  frame Enabled {
                    w8917 = 255 ("高字节1")
                  }
                }
                n3441 = Build Array(w8909, w8907) -> (w8908:i32[])
              }
              frame 6 {
                # "整组电压不均衡"
                n3442 = disable-structure shown="启用" {
                  disable-tunnel: [w8926 w8929] -> w8921
                  disable-tunnel: [w8924 w8929] -> w8919
                  disable-tunnel: w8918 -> [w8923 _]
                  frame Disabled {
                    n3443 = Unbundle By Name(w8923) -> ("整组电压不均衡"=w8922:dbl)
                    n3444 = call "输入分辨率计算-EV05.vi"("1字节?"=FALSE, "数值"=w8922, "偏移量"=0.0, "分辨率"=0.001) -> ("低字节"=w8924:dbl, "高字节1"=w8926:dbl)  [unwired: 1 in, 5 out]
                  }
                  frame Enabled {
                    w8929 = 255 ("高字节1")
                  }
                }
                n3445 = Build Array(w8921, w8919) -> (w8920:i32[])
              }
              frame 7 {
                # "单体电压过高"
                n3446 = disable-structure shown="启用" {
                  disable-tunnel: [w8938 w8941] -> w8933
                  disable-tunnel: [w8936 w8941] -> w8931
                  disable-tunnel: w8930 -> [w8935 _]
                  frame Disabled {
                    n3447 = Unbundle By Name(w8935) -> ("单体电压过高"=w8934:dbl)
                    n3448 = call "输入分辨率计算-EV05.vi"("1字节?"=FALSE, "数值"=w8934, "偏移量"=0.0, "分辨率"=0.001) -> ("低字节"=w8936:dbl, "高字节1"=w8938:dbl)  [unwired: 1 in, 5 out]
                  }
                  frame Enabled {
                    w8941 = 255 ("高字节1")
                  }
                }
                n3449 = Build Array(w8933, w8931) -> (w8932:i32[])
              }
              frame 8 {
                # "单体电压过低"
                n3450 = disable-structure shown="启用" {
                  disable-tunnel: [w8950 w8953] -> w8945
                  disable-tunnel: [w8948 w8953] -> w8943
                  disable-tunnel: w8942 -> [w8947 _]
                  frame Disabled {
                    n3451 = Unbundle By Name(w8947) -> ("单体电压过低"=w8946:dbl)
                    n3452 = call "输入分辨率计算-EV05.vi"("1字节?"=FALSE, "数值"=w8946, "偏移量"=0.0, "分辨率"=0.001) -> ("低字节"=w8948:dbl, "高字节1"=w8950:dbl)  [unwired: 1 in, 5 out]
                  }
                  frame Enabled {
                    w8953 = 255 ("高字节1")
                  }
                }
                n3453 = Build Array(w8945, w8943) -> (w8944:i32[])
              }
              frame 9 {
                # "充电电流过高"
                n3454 = disable-structure shown="启用" {
                  disable-tunnel: [w8962 w8965] -> w8957
                  disable-tunnel: [w8960 w8965] -> w8955
                  disable-tunnel: w8954 -> [w8959 _]
                  frame Disabled {
                    n3455 = Unbundle By Name(w8959) -> ("充电电流过高"=w8958:dbl)
                    n3456 = call "输入分辨率计算-EV05.vi"("1字节?"=FALSE, "数值"=w8958, "偏移量"=-3000.0, "分辨率"=0.1) -> ("低字节"=w8960:dbl, "高字节1"=w8962:dbl)  [unwired: 1 in, 5 out]
                  }
                  frame Enabled {
                    w8965 = 255 ("高字节1")
                  }
                }
                n3457 = Build Array(w8957, w8955) -> (w8956:i32[])
              }
              frame 10 {
                # "放电电流过高"
                n3458 = disable-structure shown="启用" {
                  disable-tunnel: [w8974 w8977] -> w8969
                  disable-tunnel: [w8972 w8977] -> w8967
                  disable-tunnel: w8966 -> [w8971 _]
                  frame Disabled {
                    n3459 = Unbundle By Name(w8971) -> ("放电电流过高"=w8970:dbl)
                    n3460 = call "输入分辨率计算-EV05.vi"("1字节?"=FALSE, "数值"=w8970, "偏移量"=-3000.0, "分辨率"=0.1) -> ("低字节"=w8972:dbl, "高字节1"=w8974:dbl)  [unwired: 1 in, 5 out]
                  }
                  frame Enabled {
                    w8977 = 255 ("高字节1")
                  }
                }
                n3461 = Build Array(w8969, w8967) -> (w8968:i32[])
              }
              frame 11 {
                # "单组温度不均衡"
                n3462 = disable-structure shown="启用" {
                  disable-tunnel: [w8983 255 ("高字节1")] -> w8980
                  disable-tunnel: w8978 -> [w8982 _]
                  frame Enabled {
                    n3463 = Unbundle By Name(w8982) -> ("单组温度不均衡"=w8981:dbl)
                    n3464 = call "输入分辨率计算-EV05.vi"("1字节?"=TRUE, "数值"=w8981, "分辨率"=1.0) -> ("高字节1"=w8983:dbl)  [unwired: 2 in, 6 out]
                  }
                  frame Disabled {
                  }
                }
                n3465 = Build Array(w8980) -> (w8979:dbl[])
              }
              frame 12 {
                # "SOC过高"
                n3466 = Unbundle By Name(w8991) -> ("SOC过高"=w8990:dbl)
                n3467 = call "输入分辨率计算-EV05.vi"("1字节?"=FALSE, "数值"=w8990, "偏移量"=0.0, "分辨率"=0.1) -> ("低字节"=w8992:dbl, "高字节1"=w8993:dbl)  [unwired: 1 in, 5 out]
                n3468 = call "二进制解析-8.6.vi"("索引"=4, "数值"=w8993) -> ("低位子数组"=w8996:i32[])  [unwired: 3 out]
                n3469 = call "二进制解析-8.6.vi"("索引"=4, "数值"=w8992) -> ("低位子数组"=w8988:i32[], "高位子数组"=w8995:i32[])  [unwired: 2 out]
                n3470 = Insert Into Array(array=w8996, new element=w8995) -> (w8994:i32[])  [unwired: 1 in]
                n3471 = call "数值二进制转十进制-8.6.vi"("子数组"=w8994) -> ("十进制数值"=w8989:i32)  [unwired: 4 out]
                n3472 = disable-structure shown="启用" {
                  disable-tunnel: w8989 -> [w9004 _]
                  disable-tunnel: [w9004 255 ("高字节1")] -> w8987
                  disable-tunnel: w8988 -> [w9003 _]
                  disable-tunnel: [w9003 i32[] [] ("低位子数组 29")] -> _
                  frame Disabled {
                  }
                  frame Enabled {
                  }
                }
                n3473 = Build Array(w8987, w8987) -> (w9000:i32[])
              }
              frame 13 {
                # "SOC过低"
                n3474 = Unbundle By Name(w9012) -> ("SOC过低"=w9011:dbl)
                n3475 = call "输入分辨率计算-EV05.vi"("1字节?"=FALSE, "数值"=w9011, "偏移量"=0.0, "分辨率"=0.1) -> ("低字节"=w9009:dbl, "高字节1"=w9010:dbl)  [unwired: 1 in, 5 out]
                n3476 = call "二进制解析-8.6.vi"("索引"=4, "数值"=w9010) -> ("低位子数组"=w9008:i32[])  [unwired: 3 out]
                n3477 = disable-structure shown="启用" {
                  disable-tunnel: w9009 -> [w9019 _]
                  disable-tunnel: [w9019 255 ("高字节1")] -> w9007
                  disable-tunnel: w9008 -> [w9018 _]
                  disable-tunnel: [w9018 i32[] [] ("低位子数组")] -> _
                  frame Disabled {
                    (unwired) i32[] [] ("低位子数组 4")
                  }
                  frame Enabled {
                  }
                }
                n3478 = Build Array(w9007, w9007) -> (w9015:i32[])
              }
              frame 14 {
                # "内阻过大"
                n3479 = disable-structure shown="启用" {
                  disable-tunnel: w9024 -> [w9029 _]
                  disable-tunnel: [w9025 255 ("高字节1")] -> w9022
                  frame Disabled {
                    n3480 = Unbundle By Name(w9029) -> ("内阻过大"=w9028:dbl)
                    n3481 = call "输入分辨率计算-EV05.vi"("1字节?"=TRUE, "数值"=w9028, "分辨率"=0.1) -> ("高字节1"=w9025:dbl)  [unwired: 2 in, 6 out]
                  }
                  frame Enabled {
                  }
                }
                n3482 = Build Array(w9022) -> (w9023:i32[])
              }
              frame 15 {
                # "极柱温度过高"
                n3483 = disable-structure shown="启用" {
                  disable-tunnel: w9033 -> [w9039 _]
                  disable-tunnel: [w9035 255 ("高字节1")] -> w9031
                  frame Disabled {
                    n3484 = Unbundle By Name(w9039) -> ("极柱温度过高"=w9038:dbl)
                    n3485 = call "输入分辨率计算-EV05.vi"("1字节?"=TRUE, "数值"=w9038, "偏移量"=-40.0, "分辨率"=1.0) -> ("高字节1"=w9035:dbl)  [unwired: 1 in, 6 out]
                  }
                  frame Enabled {
                  }
                }
                n3486 = Build Array(w9031) -> (w9032:i32[])
              }
              frame 16 {
                # "SOH过低"
                n3487 = disable-structure shown="启用" {
                  disable-tunnel: [w9056 w9064] -> w9043
                  disable-tunnel: w9042 -> [w9053 _]
                  disable-tunnel: [w9045 w9064] -> w9041
                  frame Disabled {
                    n3488 = Unbundle By Name(w9053) -> ("SOH过低"=w9052:dbl)
                    n3489 = call "输入分辨率计算-EV05.vi"("1字节?"=FALSE, "数值"=w9052, "偏移量"=0.0, "分辨率"=0.1) -> ("低字节"=w9054:dbl, "高字节1"=w9055:dbl)  [unwired: 1 in, 5 out]
                    n3490 = call "二进制解析-8.6.vi"("索引"=4, "数值"=w9055) -> ("低位子数组"=w9058:i32[])  [unwired: 3 out]
                    n3491 = call "二进制解析-8.6.vi"("索引"=4, "数值"=w9054) -> ("低位子数组"=w9047:i32[], "高位子数组"=w9057:i32[])  [unwired: 2 out]
                    n3492 = call "二进制解析-8.6.vi"("索引"=4, "数值"=0) -> ("低位子数组"=w9048:i32[])  [unwired: 3 out]
                    n3493 = Insert Into Array(array=w9058, new element=w9057) -> (w9051:i32[])  [unwired: 1 in]
                    n3494 = Insert Into Array(array=w9047, new element=w9048) -> (w9046:i32[])  [unwired: 1 in]
                    n3495 = call "数值二进制转十进制-8.6.vi"("子数组"=w9051) -> ("十进制数值"=w9056:i32)  [unwired: 4 out]
                    n3496 = call "数值二进制转十进制-8.6.vi"("子数组"=w9046) -> ("十进制数值"=w9045:i32)  [unwired: 4 out]
                  }
                  frame Enabled {
                    w9064 = 255 ("高字节1")
                  }
                }
                n3497 = Build Array(w9043, w9041) -> (w9044:i32[])
              }
            }
            n3498 = Insert Into Array(array=w8850, new element=w8851) -> (w8849:dbl[])  [unwired: 1 in]
          }
          n3499 = Build Array(w8846) -> (w8845:dbl[][])
          n3500 = Build Array("二级故障阀值") -> (w8836:string[])
        }
        frame "单组温度不均衡(3)" {
          n3501 = Unbundle By Name(w9070) -> ("一级故障 3"=w9071:refnum<vi>)
          n3502 = property class="Clust (严格)"(reference=w9071) -> ("Value"=w9069:T4)  [unwired: 1 in, 2 out]
          n3503 = for {
            N: 17 -> [_]
            tunnel: w9069 -> [w9081]
            shift-right: [w9078] -> w9075
            shift-left: dbl[] [] -> [w9079]
            i -> [w9082]
            n3504 = case shown="11" w9082 {
              tunnel: w9081 -> [w9083 w9094 w9105 w9115 w9125 w9135 w9147 w9159 w9171 w9183 w9195 w9207 w9220 w9241 w9253 w9262 w9271]
              tunnel: [w9084 w9095 w9106 w9116 w9126 w9137 w9149 w9161 w9173 w9185 w9197 w9208 w9229 w9244 w9252 w9261 w9273] -> w9080
              frame 0, Default {
                # "总电压过高"
                n3505 = disable-structure shown="启用" {
                  disable-tunnel: [w9090 w9093] -> w9086
                  disable-tunnel: [w9089 w9093] -> w9085
                  disable-tunnel: w9083 -> [w9088 _]
                  frame Disabled {
                    n3506 = Unbundle By Name(w9088) -> ("总电压过高"=w9087:dbl)
                    n3507 = call "输入分辨率计算-EV05.vi"("1字节?"=FALSE, "数值"=w9087, "分辨率"=0.1) -> ("低字节"=w9090:dbl, "高字节1"=w9089:dbl)  [unwired: 2 in, 5 out]
                  }
                  frame Enabled {
                    w9093 = 255 ("高字节1")
                  }
                }
                n3508 = Build Array(w9085, w9086) -> (w9084:i32[])
              }
              frame 1 {
                # "总电压过低"
                n3509 = disable-structure shown="启用" {
                  disable-tunnel: [w9101 w9104] -> w9097
                  disable-tunnel: [w9100 w9104] -> w9096
                  disable-tunnel: w9094 -> [w9099 _]
                  frame Disabled {
                    n3510 = Unbundle By Name(w9099) -> ("总电压过低"=w9098:dbl)
                    n3511 = call "输入分辨率计算-EV05.vi"("1字节?"=FALSE, "数值"=w9098, "分辨率"=0.1) -> ("低字节"=w9101:dbl, "高字节1"=w9100:dbl)  [unwired: 2 in, 5 out]
                  }
                  frame Enabled {
                    w9104 = 255 ("高字节1")
                  }
                }
                n3512 = Build Array(w9096, w9097) -> (w9095:i32[])
              }
              frame 2 {
                # "温度过高"
                n3513 = disable-structure shown="启用" {
                  disable-tunnel: [w9111 255 ("高字节1")] -> w9107
                  disable-tunnel: w9105 -> [w9109 _]
                  frame Disabled {
                    n3514 = Unbundle By Name(w9109) -> ("温度过高"=w9108:dbl)
                    n3515 = call "输入分辨率计算-EV05.vi"("1字节?"=TRUE, "数值"=w9108, "偏移量"=-40.0, "分辨率"=1.0) -> ("高字节1"=w9111:dbl)  [unwired: 1 in, 6 out]
                  }
                  frame Enabled {
                  }
                }
                n3516 = Build Array(w9107) -> (w9106:i32[])
              }
              frame 3 {
                # "温度过低"
                n3517 = disable-structure shown="启用" {
                  disable-tunnel: [w9121 255 ("高字节1")] -> w9117
                  disable-tunnel: w9115 -> [w9119 _]
                  frame Disabled {
                    n3518 = Unbundle By Name(w9119) -> ("温度过低"=w9118:dbl)
